vi "Camera Window.vi"(11 "Camera Ref":refnum<vi>) -> ()   [LabVIEW 2014]
panel:
  in  "Camera Image":T1(plugin-control)
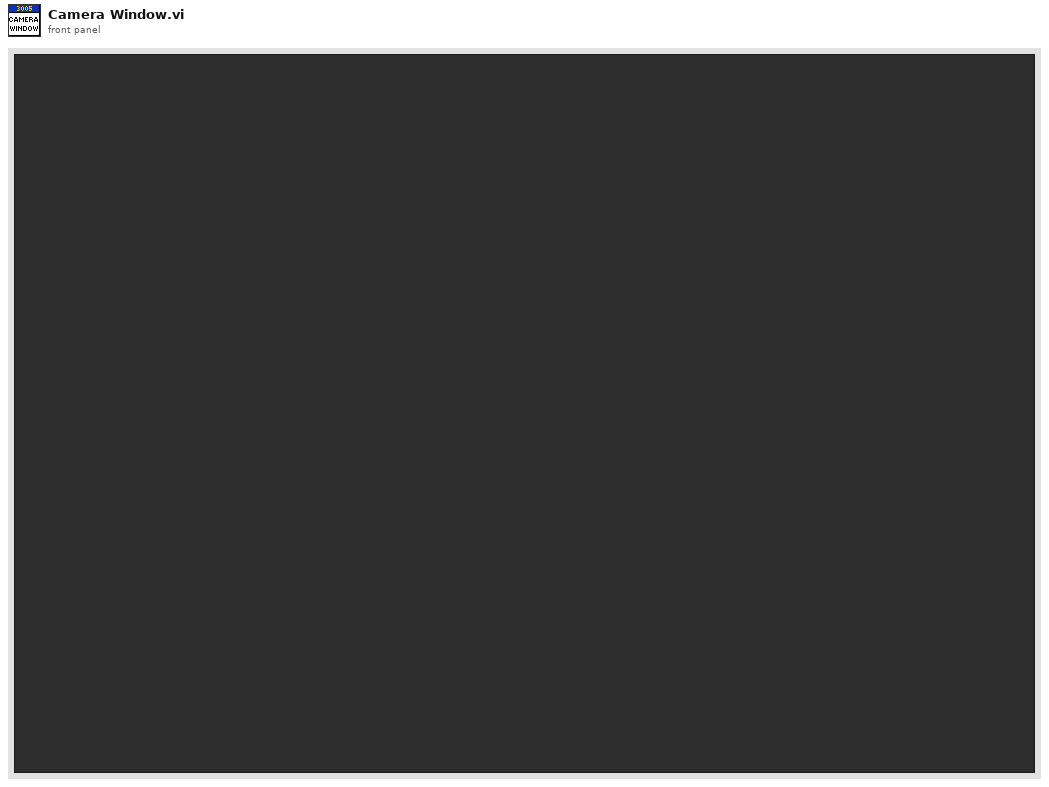
[diagram p1: front panel]
types:
  T1 = typedef "IMAQ Image.ctl" = refnum<image>
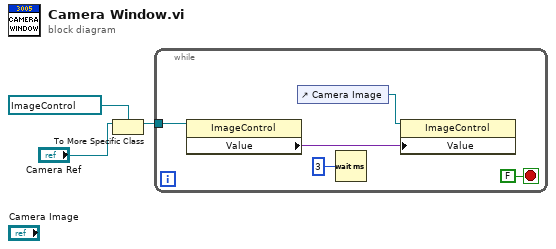
[diagram p0: block diagram]
diagram:
  n1 = To More Specific Class(target class=refnum<vi> refnum ("Camera Image"), reference="Camera Ref") -> (specific class reference=w2:refnum<vi>)  [unwired: 1 in, 1 out]
  n2 = while {
    tunnel: w2 -> [w8]
    stop <- FALSE stop-if-true
    n3 = property class="ImageControl"(reference=w8) -> ("Value"=w6:variant)  [unwired: 1 in, 2 out]
    n4 = control-ref of="Camera Image"() -> (w7:refnum<vi>)
    n5 = Wait (ms)(milliseconds to wait=u32 3) -> ()  [unwired: 1 out]
    n6 = property class="ImageControl"(reference=w7, "Value"=w6) -> ()  [unwired: 1 in, 2 out]
  }
